vi "Engage Islanding.vi"(8 "error in (no error)":errorcluster, 11 "IED in":refnum<class "IED.lvclass">) -> (0 "error out":errorcluster, 3 "IED out":refnum<class "IED.lvclass">)   [LabVIEW 2015, in "IED Actor.lvlib" / "IED.lvclass"]
uses:
  IED.lvclass
  <vilib>/ActorFramework/Actor/Actor.lvclass/Actor.ctl
  IED.lvclass/IED.ctl
  SCADA Core/SCADA Emergency Messages/Emergency Fatal Error Msg/Emergency Fatal Error Msg.lvclass/Emergency Fatal Error Msg.ctl
  <vilib>/ActorFramework/Message Enqueuer/Message Enqueuer.lvclass/Message Enqueuer.ctl
  <vilib>/NI/Tools/Keyed Array/Map String.vi
  <vilib>/ActorFramework/Message Enqueuer/Enqueue.vi
  <vilib>/NI/Tools/String/Get Case Matching.vi
  <vilib>/ActorFramework/Message Priority Queue/Priority Enqueue.vi
  SCADA Core/SCADA Emergency Messages/Emergency Fatal Error Msg/Emergency Fatal Error Msg.lvclass
  SCADA Core/SCADA Emergency Messages/Emergency Islanded Msg/Emergency Islanded Msg.lvclass
  SCADA Core/SCADA Messages/Shed Msg/Shed Msg.lvclass
  <vilib>/Modbus/master/Modbus Master.lvclass
  <vilib>/NI/Tools/Keyed Array/Tools_KeyedArray.lvlib
  Utilities/Message Strings.llb/Message String Utilities.lvlib
  <vilib>/ActorFramework/Actor/Actor.lvclass
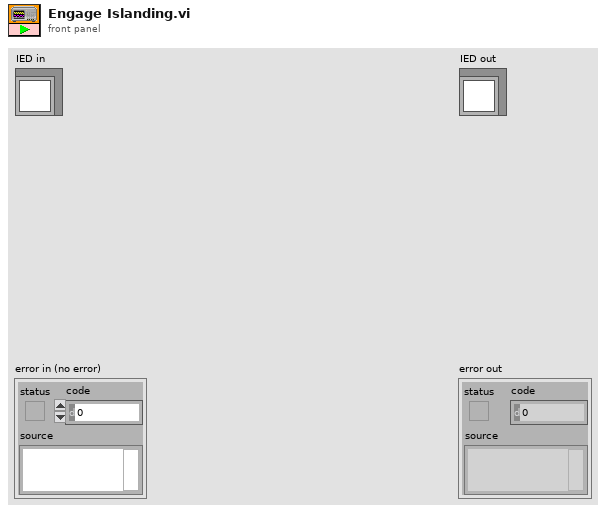
[diagram p1: front panel]
types:
  T1 = typedef "Tools_KeyedArray.lvlib/KeyedArray.ctl" = cluster{"keys":string[], "values":string[]}
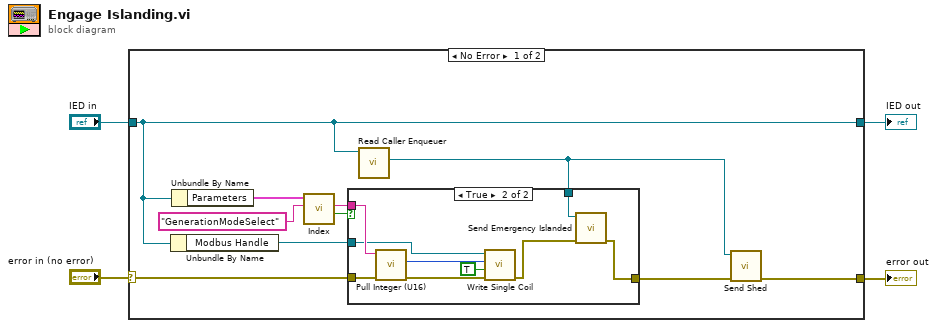
[diagram p0: block diagram]
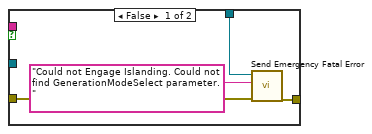
[diagram p2: hidden frame]
diagram:
  n1 = case shown="No Error" "error in (no error)" {
    selector: "error in (no error)" -> [w5 w29]
    tunnel: [w8 w29] -> w3
    tunnel: [w10 w28] -> w1
    tunnel: "IED in" -> [w10 w28]
    frame No Error {
      n2 = Unbundle By Name(w10) -> ("Modbus Handle"=w6:refnum<class "Modbus Master.lvclass">)
      n3 = Unbundle By Name(w10) -> ("Parameters"=w14:T1)
      n4 = call <vilib>:"Index.vi"("key"="GenerationModeSelect", "array in"=w14) -> ("valid key"=w11:bool, "value"=w12:string)  [unwired: 3 in, 1 out]
      n5 = call <vilib>:"Read Caller Enqueuer.vi"("Actor"=w10) -> ("Caller Enqueuer"=w9:refnum<class "Message Enqueuer.lvclass">)  [unwired: 10 in]
      n6 = case shown="True" w11 {
        tunnel: w12 -> [_ w27]
        tunnel: w5 -> [w18 w26]
        tunnel: [w17 w19] -> w7
        tunnel: w6 -> [_ w22]
        tunnel: w9 -> [w15 w21]
        frame False {
          n7 = call "Send Emergency Fatal Error.vi"("error in (no error)"=w18, "Error"="Could not Engage Islanding. Could not find GenerationModeSelect parameter.", "Message Enqueuer"=w15) -> ("error out"=w17:errorcluster)  [unwired: 7 in, 1 out]
        }
        frame True {
          n8 = call "Pull Integer (U16).vi"("error in (no error)"=w26, "String in"=w27) -> ("error out"=w25:errorcluster, "Integer out"=w24:u16)  [unwired: 7 in, 1 out]
          n9 = call-dynamic "Write Single Coil.vi"("error in (no error)"=w25, "coil value"=TRUE, "address"=w24, "Modbus master in"=w22) -> ("error out"=w20:errorcluster)  [unwired: 6 in, 1 out]
          n10 = call "Send Emergency Islanded.vi"("error in (no error)"=w20, "Message Enqueuer"=w21) -> ("error out"=w19:errorcluster)  [unwired: 8 in, 1 out]
        }
      }
      n11 = call "Send Shed.vi"("error in (no error)"=w7, "Message Enqueuer"=w9) -> ("error out"=w8:errorcluster)  [unwired: 8 in, 1 out]
    }
    frame Error {
    }
  }
  "error out" <- w3
  "IED out" <- w1
